vi "Memory.Pointer.Type Cast.Unsafe.vi"(0 "src pointer in":refnum<class "Memory.Pointer.lvclass">, 1 "dst width":u64 format="%d bytes", 2 "src width":u64 format="%d bytes", 3 "byte order (big-endian)":enum16{"big-endian", "little-endian"}(ring), 5 "dst pointer in":refnum<class "Memory.Pointer.lvclass">, 7 "src offset (0)":u64 format="%d bytes", 9 "dst offset (0)":u64 format="%d bytes", 11 "error in (no error)":errorcluster, 12 "clear dst bytes? (T)":bool=TRUE) -> (4 "src pointer out":refnum<class "Memory.Pointer.lvclass">, 6 "dst pointer out":refnum<class "Memory.Pointer.lvclass">, 15 "error out":errorcluster)   [LabVIEW 2016, in "Memory Manager.lvlib" / "Memory.Pointer.lvclass"]
doc: "Moves bytes of data from the <b>src pointer</b> at <b>src offset</b> to the <b>dst pointer</b> at <b>dst offset</b> using the <b>byte order</b> specified. <b>src width</b> and <b>dst width</b> are used to determine how many bytes to move, as well as where the bytes should be read from/written to in memory. For example, to type cast a DBL to a U16, src width would be 8 bytes and dst width would be 2 bytes.\n\nThe optional argument <b>clear dst bytes</b> will clear the subset of bytes within <b>dst pointer</b> before moving data from the <b>src pointer</b>. This is required when type casting from a smaller type to a larger type, as the larger type may have non-zero bytes that will not get overwritten. This argument can be set the FALSE when casting larger types down to smaller types.\n\n<b>Note:</b> This VI is <b>unsafe</b>, meaning it does not performs null pointer and bounds checks to prevent invalid memory access. Invalid arguments provided to this method can crash or corrupt LabVIEW memory."
uses:
  Memory.Pointer.lvclass
  Memory.Pointer.lvclass/Memory.Pointer.ctl
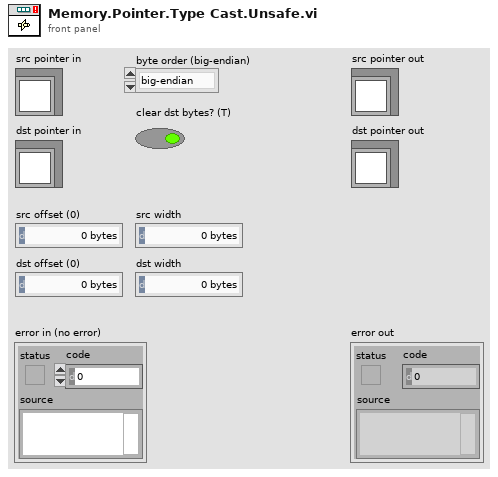
[diagram p1: front panel]
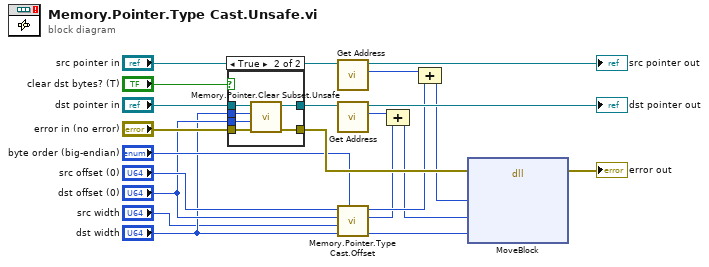
[diagram p0: block diagram]
diagram:
  n1 = case shown="True" "clear dst bytes? (T)" {
    tunnel: [w22 w29] -> w21
    tunnel: "error in (no error)" -> [w22 w28]
    tunnel: "dst pointer in" -> [w23 w27]
    tunnel: [w23 w26] -> w8
    tunnel: "dst offset (0)" -> [_ w25]
    tunnel: "dst width" -> [_ w24]
    frame False {
    }
    frame True {
      n2 = call "Memory.Pointer.Clear Subset.Unsafe.vi"("error in (no error)"=w28, "offset (0)"=w25, "length"=w24, "pointer in"=w27) -> ("error out"=w29:errorcluster, "pointer out"=w26:refnum<class "Memory.Pointer.lvclass">)  [unwired: 6 in]
    }
  }
  n3 = call "Get Address.vi"("Pointer in"="src pointer in") -> ("address"=w12:u64, "Pointer out"=→"src pointer out":refnum<class "Memory.Pointer.lvclass">)  [unwired: 8 in, 1 out]
  n4 = call "Get Address.vi"("Pointer in"=w8) -> ("address"=w7:u64, "Pointer out"=→"dst pointer out":refnum<class "Memory.Pointer.lvclass">)  [unwired: 8 in, 1 out]
  n5 = call "Memory.Pointer.Type Cast.Offset.vi"("target byte order (big-endian)"="byte order (big-endian)", "dst width"="dst width", "src width"="src width", "dst offset in"="dst offset (0)", "src offset in"="src offset (0)") -> ("bytes to move"=w14:u64, "dst offset out"=w6:u64, "src offset out"=w11:u64)  [unwired: 3 in, 1 out]
  n6 = Compound Arithmetic op=ADD(w7, w6) -> (w5:u64)
  n7 = Compound Arithmetic op=ADD(w12, w11) -> (w10:u64)
  n8 = dll-call lib="LabVIEW" fn="MoveBlock"(error in=w21, "src"=w10, "dst"=w5, "size"=w14) -> (error out=→"error out":errorcluster)  [unwired: 6 in, 1 out]
